vi "Set Item by name array.vi"(8 "error in (no error)":errorcluster, 9 "Value":refnum<class "JSON Value.lvclass">, 10 "Name Array":string[](array[string]), 11 "JSON Value In":refnum<class "JSON Value.lvclass">) -> (0 "error out":errorcluster, 1 "replaced":bool, 3 "JSON Value Out":refnum<class "JSON Value.lvclass">)   [LabVIEW 2020, in "Library Commun.lvlib" / "JSON Value.lvclass"]
doc: "Sets a JSON Value in a JSON collection by it's path. The paths is an array of strings.\nThe first element is the top level name. For elements in an array you can use a %d formatted number to index an element out.\n\nCopyright 2012 James David Powell, Shaun Rumbell and Ton Plomp\nMore information on http://lavag.org/topic/16217-cr-json-labview"
uses:
  JSON Value.lvclass
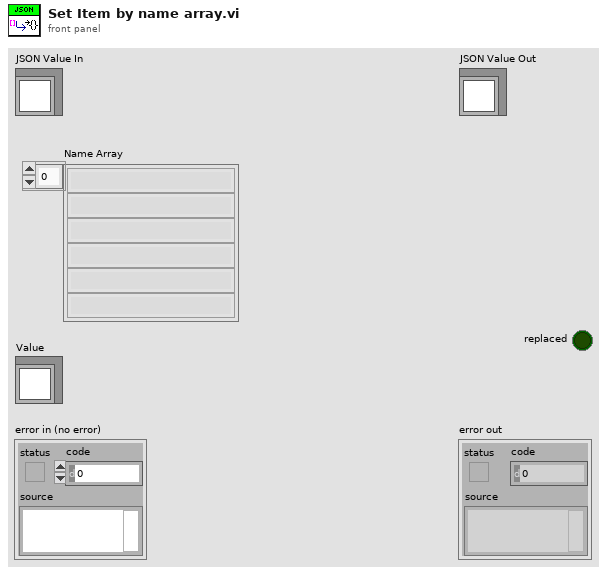
[diagram p1: front panel]
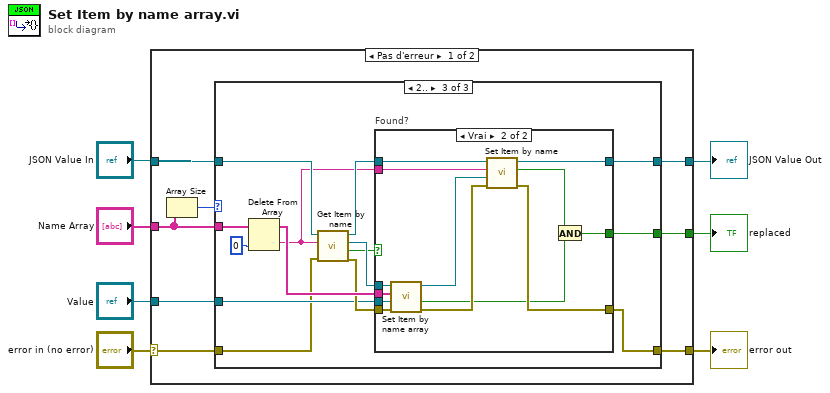
[diagram p0: block diagram]
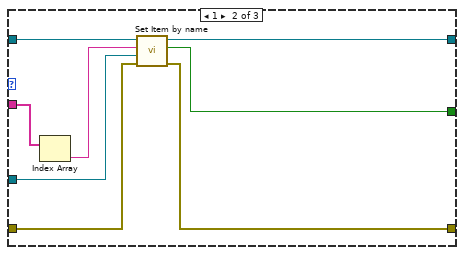
[diagram p3: hidden frame]
diagram:
  n1 = case shown="Pas d'erreur" "error in (no error)" {
    selector: "error in (no error)" -> [w9 w55]
    tunnel: [w14 w56] -> w6
    tunnel: "JSON Value In" -> [w15 w56]
    tunnel: "Name Array" -> [w12 _]
    tunnel: [w13 _] -> w3
    tunnel: "Value" -> [w10 _]
    tunnel: [w8 w55] -> w1
    frame No Error {
      n2 = Array Size(array=w12) -> (size(s)=w11:i32)
      n3 = case shown="2.." w11 {
        tunnel: w15 -> [w17 w25 w35]
        tunnel: [w17 w24 w30] -> w14
        tunnel: [_ w18 w34] -> w13
        tunnel: w12 -> [_ w23 w33]
        tunnel: w10 -> [_ w21 w32]
        tunnel: w9 -> [w16 w20 w28]
        tunnel: [w16 w19 w27] -> w8
        frame 0, Default {
        }
        frame 1 {
          n4 = Index Array(array=w23) -> (element=w22:string)  [unwired: 1 in]
          n5 = call-dynamic "Set Item by name.vi"("error in (no error)"=w20, "Value"=w21, "name"=w22, "JSON Value In"=w25) -> ("error out"=w19:errorcluster, "replaced"=w18:bool, "JSON Value Out"=w24:refnum<class "JSON Value.lvclass">)  [unwired: 5 in]
        }
        frame 2.. {
          n6 = Delete From Array(array=w33, index=0) -> (deleted portion=w29:string, array with subset deleted=w37:string[])  [unwired: 1 in]
          n7 = call-dynamic "Get Item by name.vi"("error in (no error)"=w28, "name"=w29, "JSON Value In"=w35) -> ("error out"=w36:errorcluster, "found"=w26:bool, "Value"=w38:refnum<class "JSON Value.lvclass">, "JSON Value Out"=w31:refnum<class "JSON Value.lvclass">)  [unwired: 5 in]
          n8 = case "Found?" shown="Vrai" w26 {
            tunnel: w38 -> [_ w54]
            tunnel: w37 -> [_ w53]
            tunnel: w36 -> [w41 w52]
            tunnel: [_ w42] -> w34
            tunnel: w32 -> [_ w51]
            tunnel: w31 -> [w40 w50]
            tunnel: [w40 w49] -> w30
            tunnel: w29 -> [_ w47]
            tunnel: [w41 w45] -> w27
            frame False {
            }
            frame True {
              n9 = call "Set Item by name array.vi"("error in (no error)"=w52, "Value"=w51, "Name Array"=w53, "JSON Value In"=w54) -> ("error out"=w48:errorcluster, "replaced"=w43:bool, "JSON Value Out"=w46:refnum<class "JSON Value.lvclass">)  [unwired: 5 in]
              n10 = call-dynamic "Set Item by name.vi"("error in (no error)"=w48, "Value"=w46, "name"=w47, "JSON Value In"=w50) -> ("error out"=w45:errorcluster, "replaced"=w44:bool, "JSON Value Out"=w49:refnum<class "JSON Value.lvclass">)  [unwired: 5 in]
              n11 = And(x=w44, y=w43) -> (x .and. y?=w42:bool)
            }
          }
        }
      }
    }
    frame Error {
    }
  }
  "error out" <- w1
  "JSON Value Out" <- w6
  "replaced" <- w3
